vi "Read Object Layout from Refnum.vi"(8 "error in":errorcluster, 11 "GObj refnum":refnum<vi>) -> (0 "error out":errorcluster, 2 "found?":bool, 3 "object layout":refnum<class "Object Layout.lvclass">)   [LabVIEW 2010, in "NI_SE_Front Panel Layout.lvlib"]
uses:
  NI_SE_Front Panel Layout.lvlib
  Object Layout Classes/Object Layout/Object Layout.lvclass
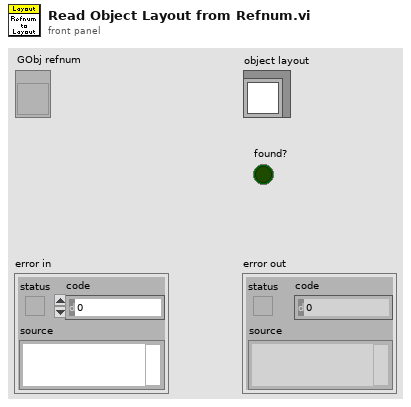
[diagram p1: front panel]
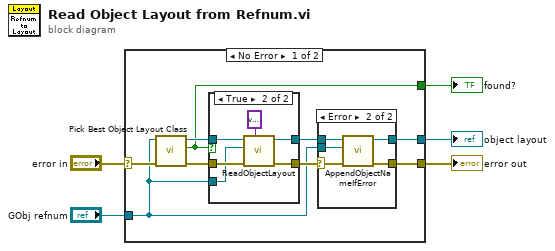
[diagram p0: block diagram]
diagram:
  n1 = case shown="No Error" "error in" {
    selector: "error in" -> [w12 w30]
    tunnel: "GObj refnum" -> [w8 _]
    tunnel: [w11 _] -> w4
    tunnel: [w6 _] -> w3
    tunnel: [w7 w30] -> w1
    frame No Error {
      n2 = call "Pick Best Object Layout Class.vi"("error in"=w12, "GObj Refnum"=w8) -> ("error out"=w14:errorcluster, "found?"=w11:bool, "object layout class"=w13:refnum<class "Object Layout.lvclass">)  [unwired: 7 in]
      n3 = case shown="True" w11 {
        tunnel: w14 -> [w22 w29]
        tunnel: w13 -> [w23 w28]
        tunnel: w8 -> [_ w27]
        tunnel: [w23 w25] -> w10
        tunnel: [w22 w26] -> w9
        frame False {
        }
        frame True {
          n4 = call-dynamic "ReadObjectLayout.vi"("properties to ignore"=variant, "error in (no error)"=w29, "GObj Refnum"=w27, "Object Layout in"=w28) -> ("error out"=w26:errorcluster, "Object Layout out"=w25:refnum<class "Object Layout.lvclass">)  [unwired: 6 in]
        }
      }
      n5 = case shown="Error" w9 {
        selector: w9 -> [w15 w18]
        tunnel: w10 -> [w16 w21]
        tunnel: [w16 w20] -> w6
        tunnel: [w15 w19] -> w7
        tunnel: w8 -> [_ w17]
        frame No Error {
        }
        frame Error {
          n6 = call-dynamic "AppendObjectNameIfError.vi"("error in (no error)"=w18, "GObj Refnum"=w17, "Object Layout in"=w21) -> ("error out"=w19:errorcluster, "Object Layout out"=w20:refnum<class "Object Layout.lvclass">)  [unwired: 7 in]
        }
      }
    }
    frame Error {
    }
  }
  "found?" <- w4
  "object layout" <- w3
  "error out" <- w1
